vi "FPGAmain_x410_IQ_PID.vi"() -> ()   [LabVIEW 2025]
uses:
  FPGA/DataMode.ctl
  FPGA/Input_5782/5782_Fast_PID_states.ctl
  <vilib>/Platform/TimedLoop/XDataNode/timing_clust.ctl
  <vilib>/Platform/TimedLoop/XDataNode/nitl_modes.ctl
  <vilib>/Platform/TimedLoop/XDataNode/wakeup.ctl
  <vilib>/rvi/Emulation/niFpgaSctlEmulationGetInTimedLoop.vi
  <vilib>/rvi/Emulation/niFpgaEmulationReportErrorSimple.vi
  <vilib>/rvi/Emulation/niFpgaGetClockAttributes.vi
  <vilib>/rvi/Emulation/niFpgaCriticalErrorInLSC.vi
  <vilib>/rvi/Emulation/niFpgaEmulationIsFPGAContextNoSignature.vi
  <vilib>/rvi/DataTransferAndStorage/Container/Common/niFpgaContainerGetUniqueNameForEmu.vi
  <vilib>/rvi/Memory/Memory_Emulation/niFpgaMemoryEmulationCacheClearOnFirstRun.vi
  <vilib>/rvi/Memory/Memory_Emulation/nirvimemoryEmulationManagerCache_MakeExclusive.vi
  <vilib>/rvi/Memory/Memory_Emulation/niFpgaMemoryEmulationValidateCache.vi
  <vilib>/rvi/Memory/Memory_Emulation/nirvimemoryEmulationManagerCache_InsertValue.vi
  <vilib>/Utility/error.llb/Clear Errors.vi
  <vilib>/rvi/Memory/Memory_Emulation/nirvimemoryEmulationManagerCache_ReleaseExclusive.vi
  <vilib>/rvi/Memory/Memory_Emulation/nirvimemoryEmulationManagerCache_GetValue.vi
  <vilib>/rvi/Memory/Memory_Emulation/nirvimemoryEmulationManagerCache_SetValue.vi
  <vilib>/rvi/Emulation/niFpgaProcessEmulError.vi
  <vilib>/rvi/errors/niFpgaSetErrorForExecOnDevCompSimple.vi
  <vilib>/rvi/eio/common/nirviEmuReportErrorAndStop.vi
  <vilib>/rvi/FIFO/Fifo_Resource/nirvififoEmulationSetSize.vi
  <vilib>/rvi/FIFO/Fifo_Resource/nirviFifoEmulationQueueMgr.vi
  <instcachedir>/0/nirviFifoEmulationQueueMgr_E5CAEC123FF24DC58D834DCA3CDAA9B5.lvgen/nirviFifoEmulationQueueMgr_E5CAEC123FF24DC58D834DCA3CDAA9B5_017.vi
  <vilib>/rvi/FIFO/Fifo_Resource/nirvififoEmulationCreateLock.vi
  <vilib>/rvi/FIFO/Fifo_Resource/nirvififoEmulationObtainLock.vi
  <vilib>/rvi/FIFO/Fifo_Resource/nirvififoEmulationReleaseLock.vi
  <vilib>/rvi/occurrence/nirviWaitOnOccurrenceBase.vi
  <vilib>/rvi/errors/nirviReportUnexpectedCaseInternalError.vi
  <vilib>/rvi/errors/nirviReportUnexpectedCaseInternalError (U32).vi
  <instcachedir>/0/nirviFifoEmulationQueueMgr_E5CAEC123FF24DC58D834DCA3CDAA9B5.lvgen/nirviFifoEmulationQueueMgr_E5CAEC123FF24DC58D834DCA3CDAA9B5_004.vi
  <vilib>/rvi/FIFO/Fifo_Resource/nirvififoEmulationDetermineInputValidOut.vi
  <instcachedir>/0/nirviFifoEmulationQueueMgr_E5CAEC123FF24DC58D834DCA3CDAA9B5.lvgen/nirviFifoEmulationQueueMgr_E5CAEC123FF24DC58D834DCA3CDAA9B5_016.vi
  <vilib>/eio/utilities/niEioResolveVilibRelativePath.vi
  <vilib>/rvi/interface/RandomDataEmulation/niFpgaRandomDataHandleErrors.vi
  <instcachedir>/0/nirviFifoEmulationQueueMgr_E5CAEC123FF24DC58D834DCA3CDAA9B5.lvgen/nirviFifoEmulationQueueMgr_E5CAEC123FF24DC58D834DCA3CDAA9B5_006.vi
  <vilib>/rvi/interface/RandomDataEmulation/nirviRandomDataMultiElementFPGAFIFO.vi
  <instcachedir>/0/nirviRandomDataMultiElementFPGAFIFO_BE2FF10D3D6E420AB0291A02835C249E.lvgen/nirviRandomDataMultiElementFPGAFIFO_BE2FF10D3D6E420AB0291A02835C249E_001.vi
  <vilib>/Platform/TimedLoop/XDataNode/XDataNode.xnode
  <vilib>/rvi/DataTransferAndStorage/Container/XNode/niFpgaContainer.xnode
  <vilib>/rvi/DataTransferAndStorage/Register/Emulation/niFpgaRegisterEmulation.vi
  <vilib>/rvi/FIFO/Fifo_Resource/nirvififoEmulationRead.vi
  <vilib>/rvi/FIFO/Fifo_Resource/nirvififoEmulationWrite.vi
  <vilib>/rvi/interface/RandomDataEmulation/nirviRandomDataFpgaReadWriteTemplate.vi
  <vilib>/rvi/interface/RandomDataEmulation/nirviRandomDataFpgaMultiElementTemplate.vi
  <vilib>/eio/EIONode/EIONode.xnode
  <vilib>/rvi/eio/common/nirviEmuTemplateMethod_errors.vi
  <vilib>/Platform/TimedLoop/XDataNode/XDNodeRunTimeDep.lvlib
  <instrlib>/_niInstr/Basic Elements/v1/FPGA/niInstr Basic Elements v1 FPGA.lvlib
panel:
  in  "Output gain":fxp<+/-,16,10>
  out "Amp1":fxp<+,16,14>
  out "TaM":fxp<+/-,32,13>
  out "Quench_Warning":bool
  out "Tau_set":fxp<+/-,32,13>
  in  "Ultra low speed transfer":bool
  out "5782 states":T1
  in  "Full speed transfer":bool
  in  "IO Module\\AO Data Sync":bool=TRUE
  in  "IO Module\\SPI Write Data":u16
  out "IO Module\\SPI Read Data":u8
  in  "IO Module\\SPI Read":bool
  in  "IO Module\\SPI Write":bool
  in  "IO Module\\SPI Address":u16
  in  "IO Module\\SPI Device":u8
  out "IO Module\\SPI Idle":bool
  in  "AM phase":fxp<+,64,64>
  in  "User Command Commit":bool
  in  "User Command":u8
  out "User Command Idle":bool
  out "User Command Status":u8
  in  "User Data 0":u8
  in  "User Data 1":u8
  out "PLL Locked":bool
  out "User Error":bool
  out "Configured?":bool
  in  "Continuous":bool
  in  "Record length":u16=4000 caption="Samples Per Trigger" min=1 step=1
  in  "Trigger Acquisition":bool
  out "IO Module\\Trigger Input":bool
  in  "Acquisition running":bool
  in  "Phase output":fxp<+,64,64>[](array[numeric])=[0.0, 0.0, 0.0, 0.0]
  in  "Simulated phase":fxp<+,64,64>[](array[numeric])=[0.0, 0.0]
  in  "Mode":T2
  in  "Phase input":fxp<+,64,64>[](array[numeric])=[0.0, 0.0, 0.0, 0.0, 0.0, 0.0, 0.0, 0.0, 0.0, 0.0, 0.0, 0.0, 0.0, 0.0, 0.0, 0.0]
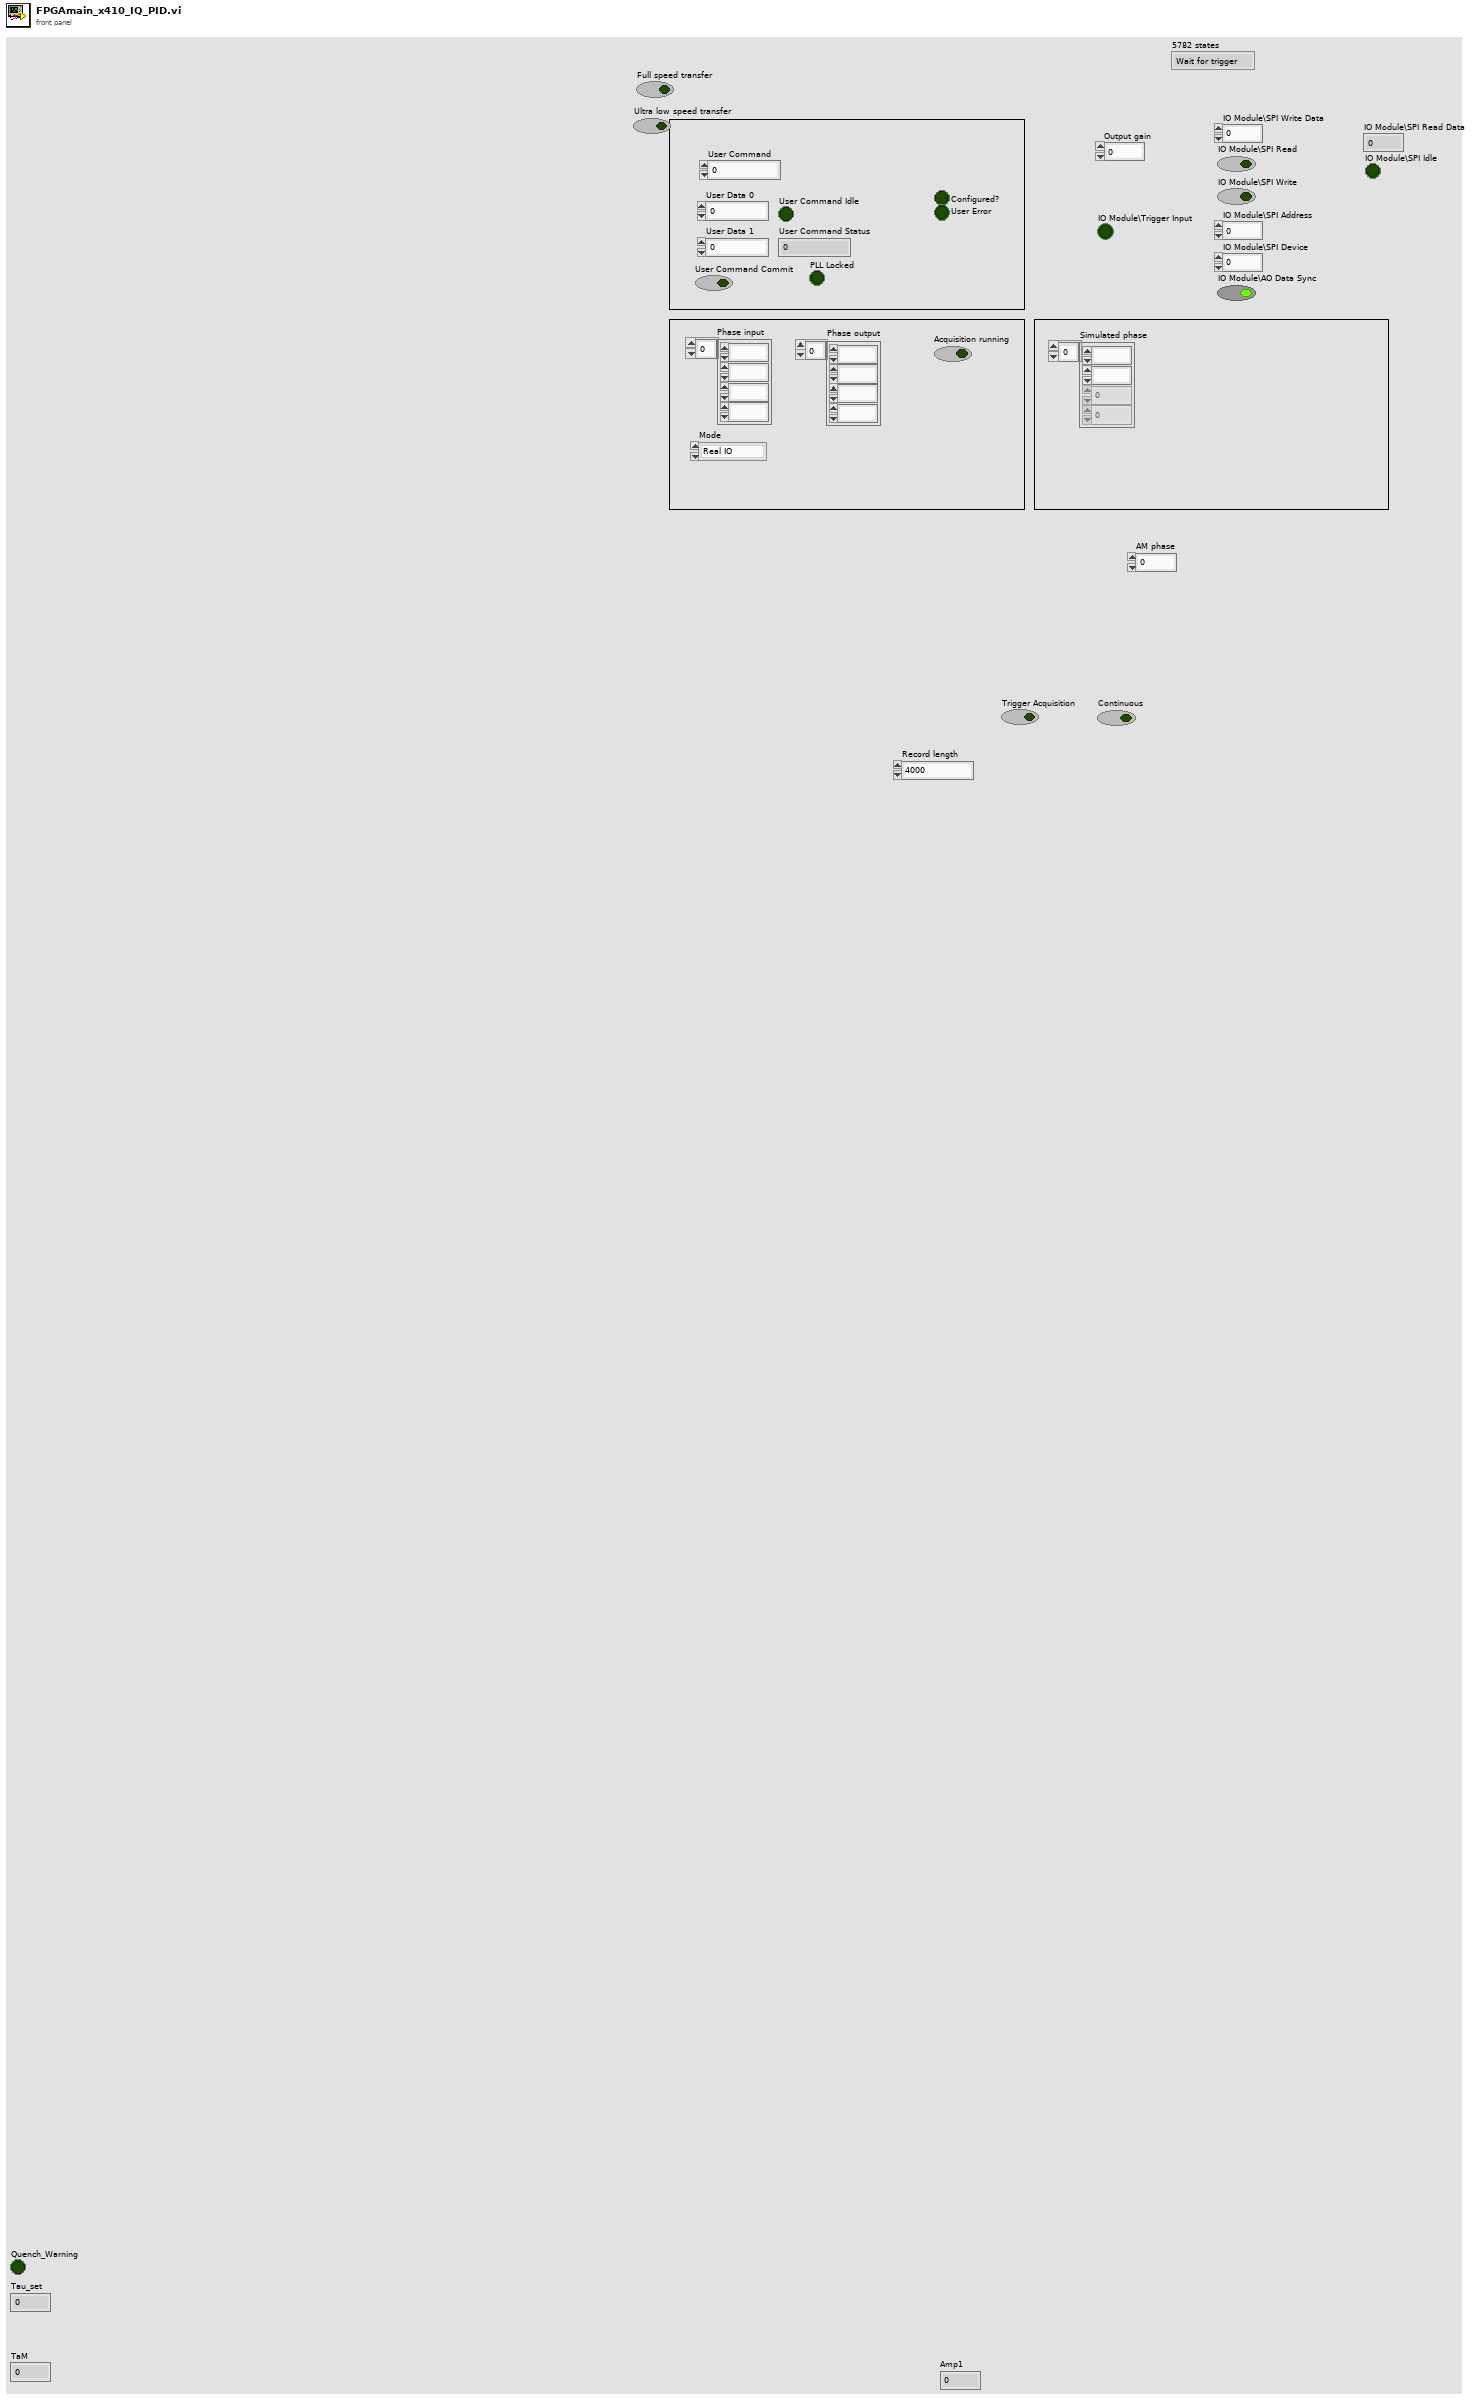
[diagram p1: front panel]
types:
  T1 = typedef "5782_Fast_PID_states.ctl" = enum8{"Wait for trigger", "Acquisition", "Send record length", "Wait for output", "Quiet period"}
  T2 = typedef "DataMode.ctl" = enum16{"Real IO", "Simulated"}
  T3 = typedef "XDNodeRunTimeDep.lvlib/timing_clust.ctl" = cluster{"Expected End [f-1]":u64, "Actual End [f-1]":u64, "Finished Late? [f-1]":bool, "Expected End [i-1]":u64, "Actual End [i-1]":u64, "Finished Late? [i-1]":bool, "Expected Start [i]":u64, "Actual Start [i]":u64, "Expected Start [f]":u64, "Actual Start [f]":u64, "Source Name":string, "Structure Name":string, "Period":i64, "Deadline":i64, "Offset":i64, "Start":i64, "Priority":i32, "Timeout":i32, "Mode":T4, "Wakeup Reason":T5, "Error":errorcluster, "Source Type":string, "Secondary Source Type":string, "Global End Time":u64, "Global Start Time":u64, "Frame Duration":u64, "Iteration Duration":u64, "Assigned CPU":i32, "I/O Scan Engine Mode":u32}
  T4 = typedef "XDNodeRunTimeDep.lvlib/nitl_modes.ctl" = enum32{"No Change", "Process missed periods, maintain original phase", "Discard missed periods, maintain original phase", "Process missed periods, ignore original phase", "Discard missed periods, ignore original phase"}
  T5 = typedef "XDNodeRunTimeDep.lvlib/wakeup.ctl" = enum32{"Normal", "Aborted", "Asynchronous wakeup", "Timing source error", "Timed loop error", "Timeout"}
  T6 = typedef "niInstr DSP v1 Shared.lvlib/IQ Data.ctl" = cluster{"I":fxp<+/-,18,1>, "Q":fxp<+/-,18,1>, "overflow":bool}
  T7 = cluster{"I":fxp<+/-,18,1>, "Q":fxp<+/-,18,1>, "overflow":bool}
  T8 = cluster{"I":fxp<+/-,18,1>, "Q":fxp<+/-,18,1>, "overflow":bool}[]
  T9 = typedef "I32 array size 4.ctl" = fxp<+/-,32,14>[]
  T10 = typedef "IQ-1element.ctl" = T6[]
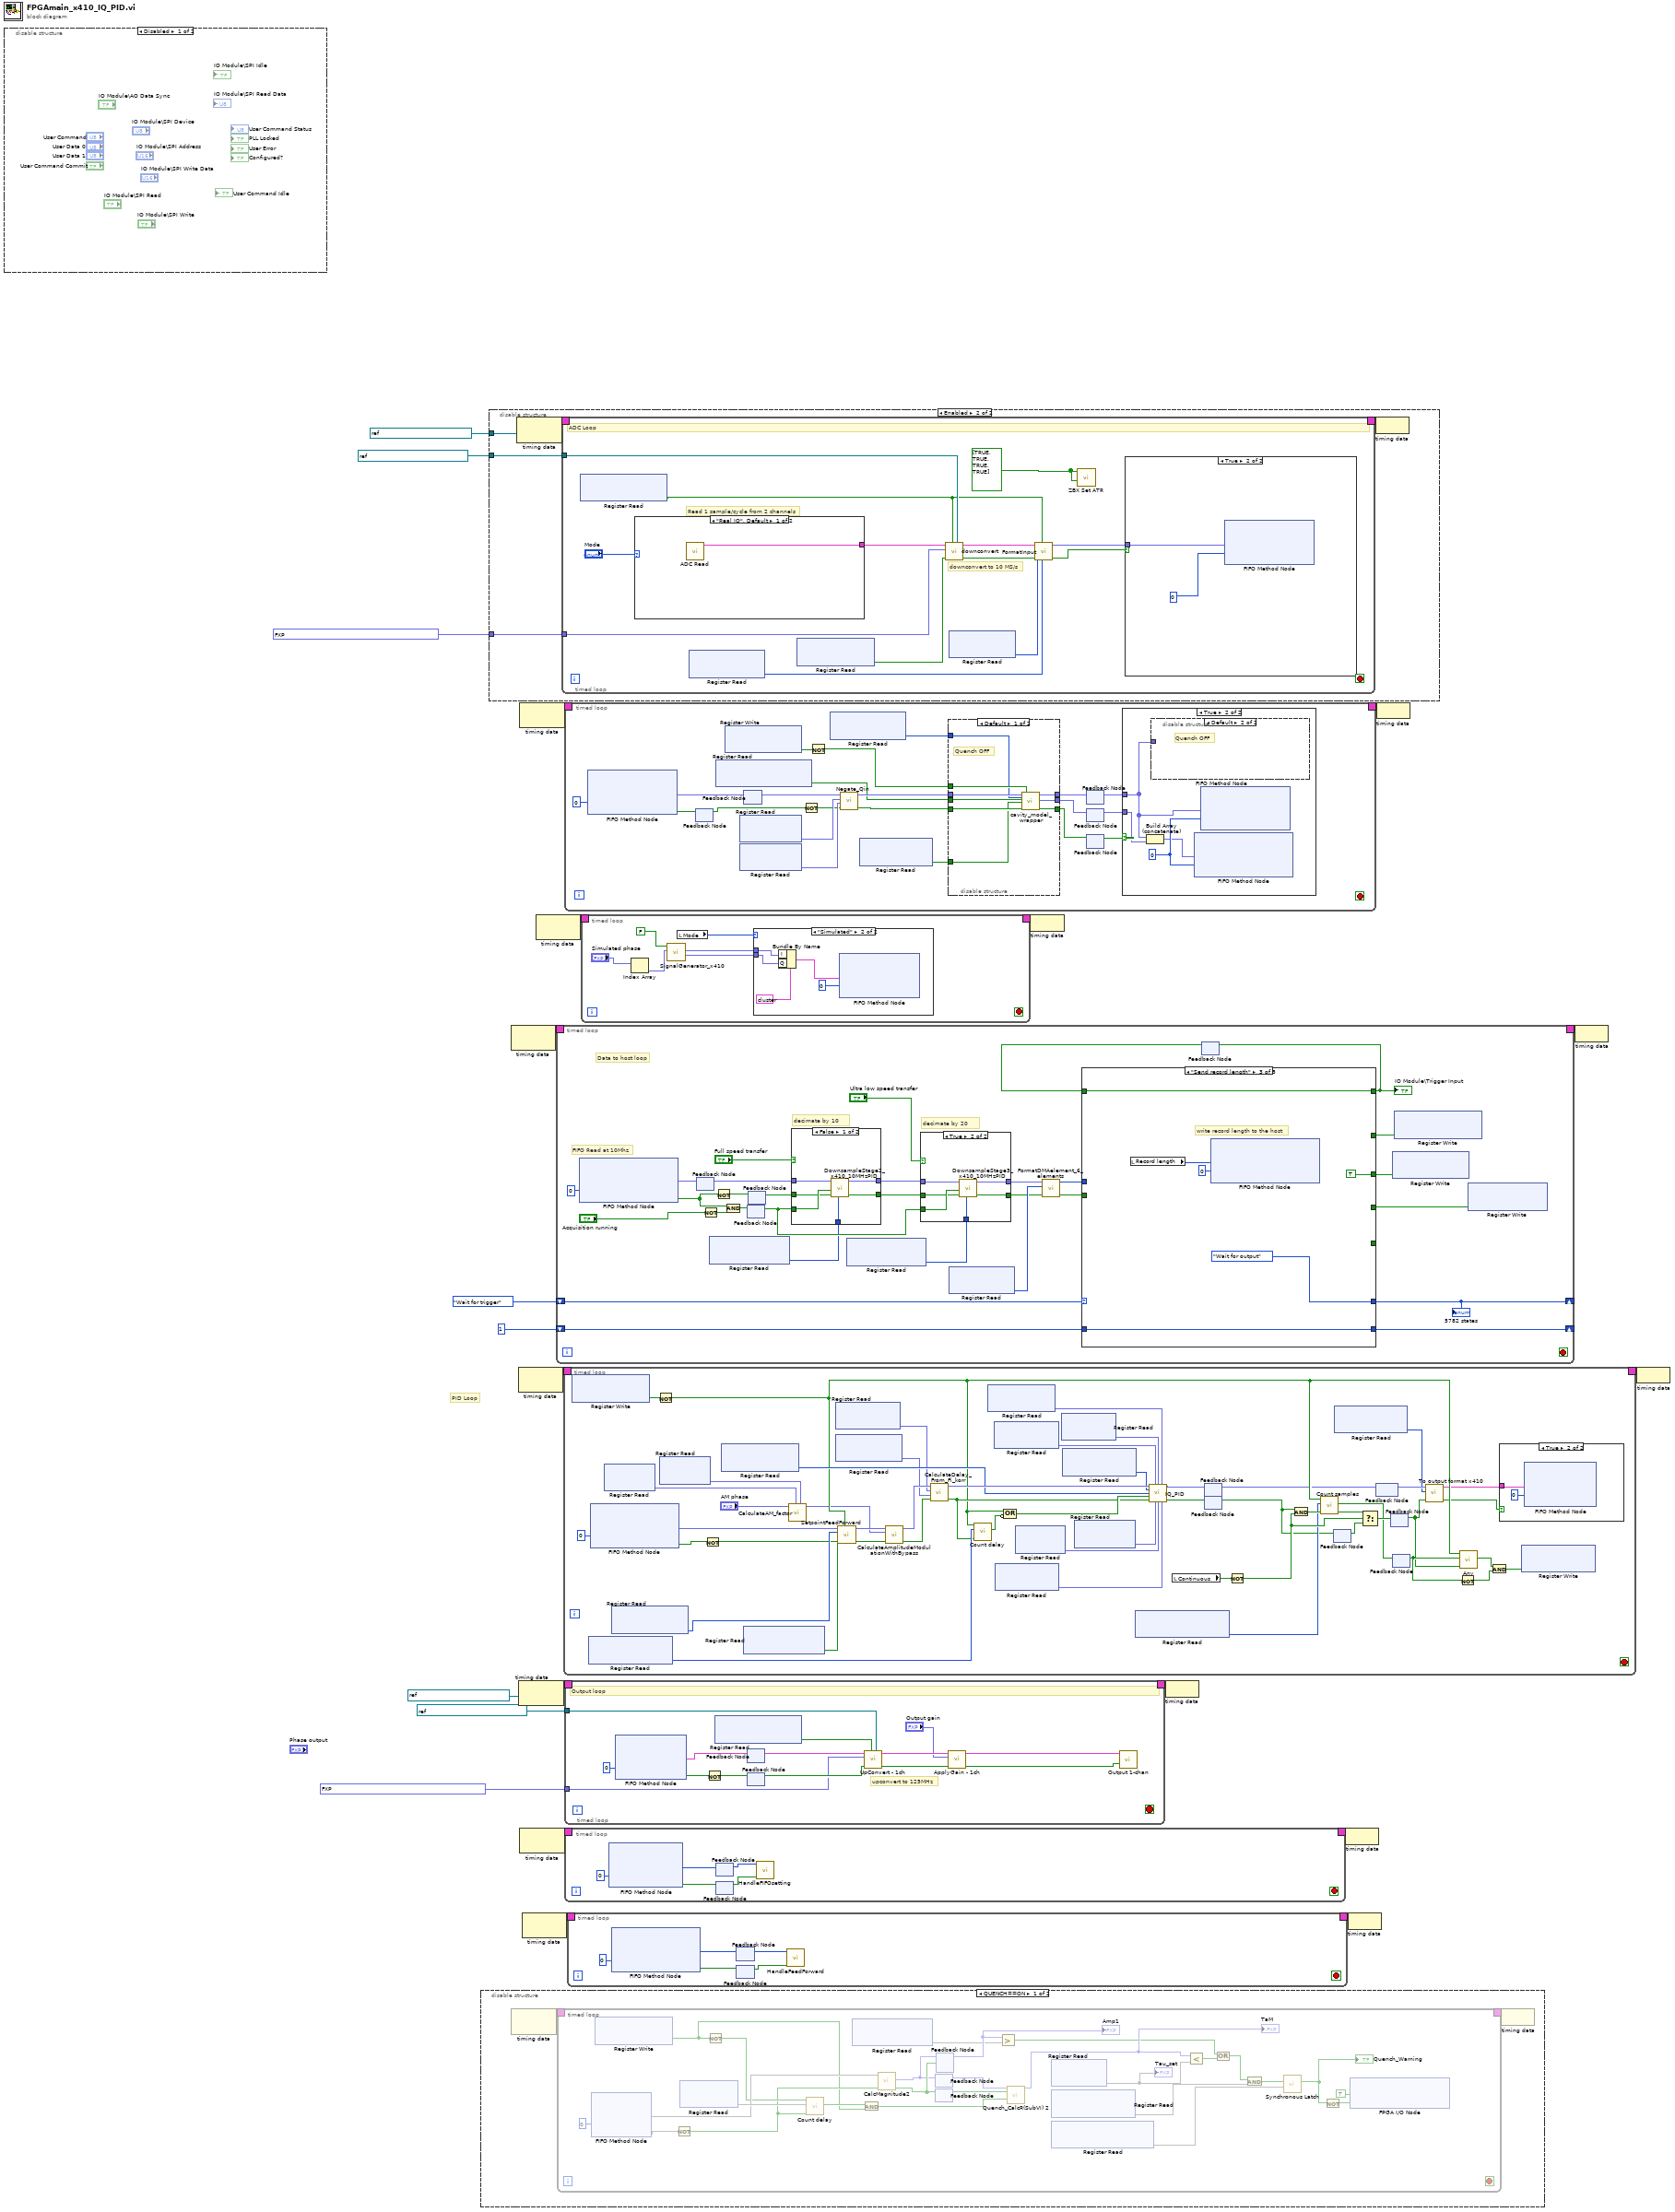
[diagram p0: block diagram]
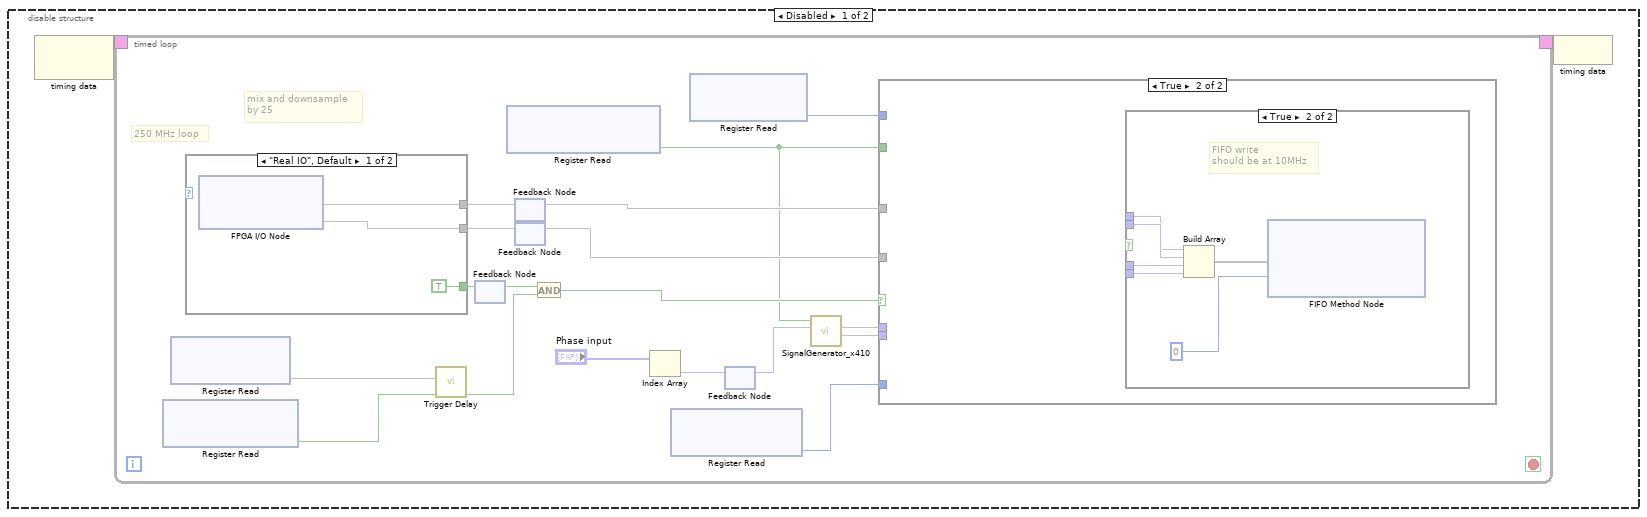
[diagram p2: hidden frame]
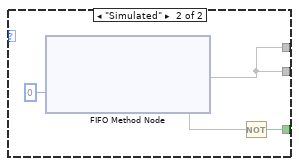
[diagram p5: hidden frame]
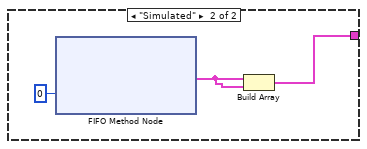
[diagram p6: hidden frame]
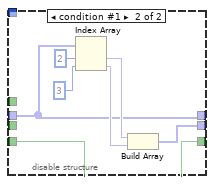
[diagram p11: hidden frame]
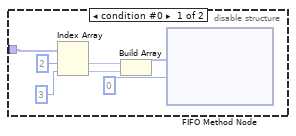
[diagram p13: hidden frame]
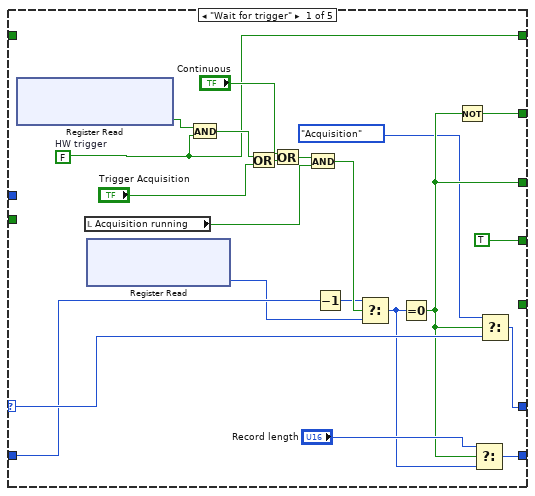
[diagram p16: hidden frame]
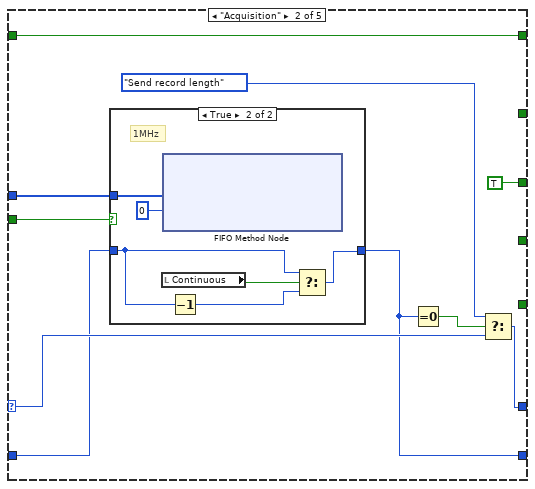
[diagram p17: hidden frame]
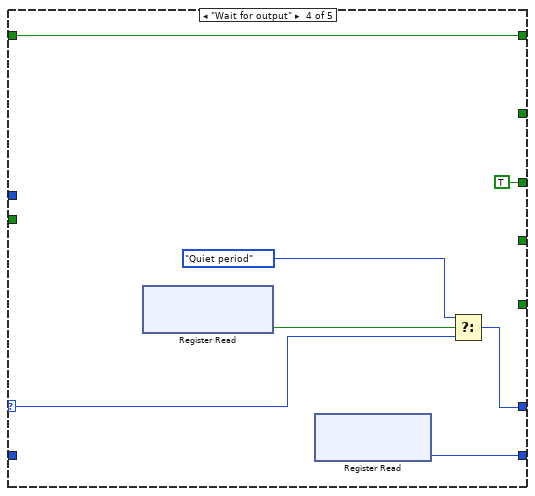
[diagram p19: hidden frame]
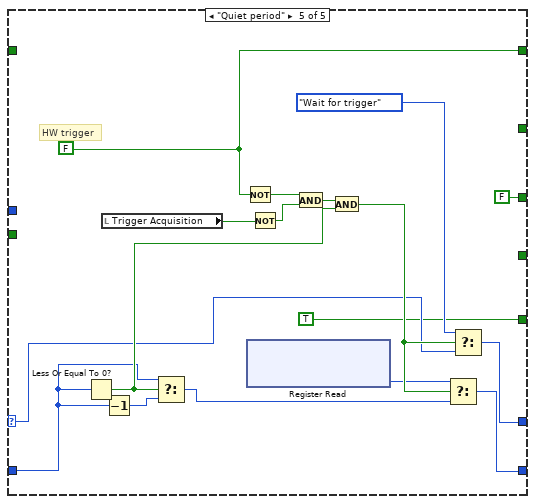
[diagram p20: hidden frame]
diagram:
  # "PID Loop"
  n1 = disable-structure shown="Disabled" {
    frame Disabled {
    }
    frame Enabled {
    }
  }
  n2 = disable-structure shown="QUENCH==ON" {
    frame condition #0 {
      n3 = node-c288() -> (w24:T3)  [unwired: 1 in]
      n4 = timed-loop {
        timing: w24 -> [_]
        timing-out: [_] -> w23
        stop <- _ stop-if-true
        n5 = xnode ("FIFO Method Node")("Timeout"=0) -> ("Element"=w40, "Timed Out?"=w38)  [unwired: 1 in, 1 out]
        n6 = xnode ("Register Write")() -> ("Data"=w34:bool)  [unwired: 1 in, 1 out]
        n7 = Not(x=w38) -> (.not. x?=w37:bool)
        n8 = xnode ("Register Read")() -> ("Data"=w41)  [unwired: 1 in, 1 out]
        n9 = Not(x=w34) -> (.not. x?=w39:bool)
        n10 = call "Count delay.vi"("input valid"=w37, "Count to skip"=w41, "Reset"=w39) -> ("count done?"=w45:bool)  [unwired: 7 in, 1 out]
        n11 = xnode "Register Read"() -> ("Data"=w28)  [unwired: 1 in, 1 out]
        n12 = And(x=w45, y=w34) -> (x .and. y?=w42:bool)
        n13 = call "CalcMagnitude2.vi"("input valid"=w37, "Data in"=w40) -> ("output valid"=w30:bool, "Amp1"=w29:fxp<+,16,14>)  [unwired: 8 in]
        n14 = feedback #1() -> (w44:fxp<+,16,14>)  [unwired: 1 in]
        n15 = feedback-in #1(w29) -> ()
        n16 = feedback #2() -> (w43:bool)  [unwired: 1 in]
        n17 = feedback-in #2(w30) -> ()
        n18 = feedback #3() -> (w31:fxp<+,16,14>)  [unwired: 1 in]
        "Amp1" <- w31
        n19 = feedback-in #3(w29, w30) -> ()
        n20 = Greater?(x=w31, y=w28) -> (0:w25:bool)
        n21 = call "Quench_CalcR(SubVI) 2.vi"("Mag"=w44, "input valid"=w43, "count done?"=w42) -> ("Tau meas"=w35:fxp<+/-,32,13>)  [unwired: 12 in]
        "TaM" <- w35
        n22 = xnode ("Register Read")() -> ("Data"=w49)  [unwired: 1 in, 1 out]
        n23 = xnode ("Register Read")() -> ("Data"=w47)  [unwired: 1 in, 1 out]
        "Tau_set" <- w47
        n24 = xnode ("Register Read")() -> ("Data"=w50)  [unwired: 1 in, 1 out]
        n25 = Less?(x=w35, y=w47) -> (x < y?=w27:bool)
        n26 = Or(x=w25, y=w27) -> (x .or. y?=w26:bool)
        n27 = And(x=w26, y=w50) -> (x .and. y?=w48:bool)
        n28 = call <instrlib>:"Synchronous Latch.vi"("clear"=w49, "set"=w48) -> ("out"=w46:bool)  [unwired: 9 in]
        "Quench_Warning" <- w46
        n29 = Not(x=w46) -> (.not. x?=w33:bool)
        n30 = xnode "FPGA I/O Node"("IO Module\\PFI 2 WE"=TRUE ("IO Module\\PFI 2 WE"), "IO Module\\PFI 2 Wr Data"=w33) -> ()  [unwired: 2 in, 2 out]
      }
      n31 = node-c288(w23) -> ()
    }
    frame condition #1 (active) {
    }
  }
  n32 = disable-structure shown="Enabled" {
    disable-tunnel: fxp<+,48,1> 0.0799999999999983 ("output sample rate") -> [_ w106]
    disable-tunnel: refnum<k21> "Daughterboard 0\\Data Clock x2" ("clock x2") -> [_ w105]
    disable-tunnel: refnum<k21> "Daughterboard 0\\Data Clock" ("Source Name") -> [_ w104]
    frame Disabled {
      n33 = node-c288() -> (w56:T3)  [unwired: 1 in]
      n34 = timed-loop {
        timing: w56 -> [_]
        timing-out: [_] -> w55
        stop <- _ stop-if-true
        # "mix and downsample\nby 25"
        # "250 MHz loop"
        n35 = xnode ("Register Read")() -> ("Data"=w62:bool)  [unwired: 1 in, 1 out]
        n36 = xnode ("Register Read")() -> ("Data"=w60)  [unwired: 1 in, 1 out]
        n37 = case shown="\"Real IO\", Default" {
          selector: _ -> [_ _]
          tunnel: [w95 w96] -> w74
          tunnel: [w94 w96] -> w72
          tunnel: [TRUE w97] -> w70
          frame "Real IO", Default {
            n38 = xnode "FPGA I/O Node"() -> ("IO Module\\AI 0"=w95, "IO Module\\AI 1"=w94)  [unwired: 2 in, 2 out]
          }
          frame "Simulated" {
            n39 = xnode ("FIFO Method Node")("Timeout"=0) -> ("Element"=w96, "Timed Out?"=w98)  [unwired: 1 in, 1 out]
            n40 = Not(x=w98) -> (.not. x?=w97:bool)
          }
        }
        n41 = call "Trigger Delay.vi"("input valid"=w62, "Count to skip"=w60) -> ("output valid"=w61:bool)  [unwired: 9 in]
        n42 = feedback #4() -> (w69:bool)  [unwired: 1 in]
        n43 = feedback-in #4(w70) -> ()
        n44 = xnode ("Register Read")() -> ("Data"=w58:bool)  [unwired: 1 in, 1 out]
        n45 = feedback #5() -> (w73)  [unwired: 1 in]
        n46 = feedback-in #5(w74) -> ()
        n47 = feedback #6() -> (w71)  [unwired: 1 in]
        n48 = feedback-in #6(w72) -> ()
        n49 = And(x=w69, y=w61) -> (x .and. y?=w66:bool)
        n50 = Index Array(array="Phase input") -> (element=w64:fxp<+,64,64>)  [unwired: 1 in]
        n51 = xnode ("Register Read")() -> ("Data"=w57:u32)  [unwired: 1 in, 1 out]
        n52 = xnode ("Register Read")() -> ("Data"=w59:u16)  [unwired: 1 in, 1 out]
        n53 = feedback #7() -> (w63:fxp<+,64,64>)  [unwired: 1 in]
        n54 = feedback-in #7(w64) -> ()
        n55 = call "SignalGenerator_x410.vi"("phase"=w63, "Reset"=w58) -> ("Cos"=w68:fxp<+/-,18,1>, "Sin"=w67:fxp<+/-,18,1>)  [unwired: 7 in, 1 out]
        n56 = case shown="True" w66 {
          tunnel: w73 -> [_ w86]
          tunnel: w71 -> [_ w85]
          tunnel: w68 -> [_ w79]
          tunnel: w67 -> [_ w78]
          tunnel: w59 -> [_ w77]
          tunnel: w58 -> [_ w76]
          tunnel: w57 -> [_ w75]
          frame False {
          }
          frame True {
            n57 = case shown="True" w82 {
              tunnel: [_ w92] -> w83
              tunnel: [_ w91] -> w84
              tunnel: [_ w90] -> w81
              tunnel: [_ w89] -> w80
              frame False {
              }
              frame True {
                # "FIFO write\nshould be at 10MHz"
                n58 = Build Array(w91, w92, w90, w89) -> (w88:void[])
                n59 = xnode ("FIFO Method Node")("Element"=w88, "Timeout"=0) -> ()  [unwired: 1 in, 2 out]
              }
            }
          }
        }
      }
      n60 = node-c288(w55) -> ()
    }
    frame Enabled {
      n61 = node-c288(w104) -> (w108:T3)
      n62 = timed-loop "Acquisition Loop" {
        timing: w108 -> [_]
        timing-out: [_] -> w107
        tunnel: w106 -> [w121]
        tunnel: w105 -> [w118]
        stop <- _ stop-if-true
        w119 = bool[] [TRUE, TRUE, TRUE, TRUE] ("DB 0")
        # "Read 1 sample/cycle from 2 channels"
        # "downconvert to 10 MS/s"
        # "ADC Loop"
        n63 = xnode ("Register Read")() -> ("Data"=w113:bool)  [unwired: 1 in, 1 out]
        n64 = case shown="\"Real IO\", Default" "Mode" {
          tunnel: [w122 w124] -> w120
          frame "Real IO", Default {
            n65 = call "ADC Read.vi"() -> ("Data out"=w122:T6[])  [unwired: 11 in]
          }
          frame "Simulated" {
            n66 = xnode ("FIFO Method Node")("Timeout"=0) -> ("Element"=w125:T7)  [unwired: 1 in, 2 out]
            n67 = Build Array(w125, w125) -> (w124:T8)
          }
        }
        n68 = xnode ("Register Read")() -> ("Data"=w114:u32)  [unwired: 1 in, 1 out]
        n69 = xnode ("Register Read")() -> ("Data"=w112:bool)  [unwired: 1 in, 1 out]
        n70 = call "downconvert.vi"("clock x2"=w118, "reset"=w113, "input valid"=w112, "output sample rate"=w121, "data in"=w120) -> ("output valid"=w111:bool, "data out"=w116:T6[])  [unwired: 5 in]
        n71 = xnode ("Register Read")() -> ("Data"=w109:u16)  [unwired: 1 in, 1 out]
        n72 = call "FormatInput.vi"("Count to skip"=w114, "reset"=w113, "valid in"=w111, "factor"=w109, "data in"=w116) -> ("valid out"=w110:bool, "Array out"=w115:T9)  [unwired: 5 in]
        n73 = call <instrlib>:"ZBX Set ATR.vi"("DB 1"=w119, "DB 0"=w119) -> ()  [unwired: 10 in]
        n74 = case shown="True" w110 {
          tunnel: w115 -> [_ w126]
          frame False {
          }
          frame True {
            n75 = xnode ("FIFO Method Node")("Element"=w126, "Timeout"=0) -> ()  [unwired: 1 in, 2 out]
          }
        }
      }
      n76 = node-c288(w107) -> ()
    }
  }
  n77 = node-c288() -> (w17:T3)  [unwired: 1 in]
  n78 = node-c288() -> (w19:T3)  [unwired: 1 in]
  n79 = node-c288(refnum<k21> "Daughterboard 0\\Data Clock" ("Source Name")) -> (w5:T3)
  n80 = node-c288() -> (w12:T3)  [unwired: 1 in]
  n81 = node-c288() -> (w21:T3)  [unwired: 1 in]
  n82 = node-c288() -> (w14:T3)  [unwired: 1 in]
  n83 = node-c288() -> (w10:T3)  [unwired: 1 in]
  n84 = timed-loop {
    timing: w17 -> [_]
    timing-out: [_] -> w16
    shift-right: [w161] -> _
    shift-left: 5782_Fast_PID_states."Wait for trigger" ("5782 states") -> [w163]
    shift-right: [w160] -> _
    shift-left: u16 1 ("trigger samples") -> [w162]
    stop <- _ stop-if-true
    # "decimate by 20"
    # "Data to host loop"
    # "FIFO Read at 10Mhz"
    # "decimate by 10"
    n85 = xnode ("FIFO Method Node")("Timeout"=0) -> ("Element"=w144:fxp<+/-,32,14>[], "Timed Out?"=w143:bool)  [unwired: 1 in, 1 out]
    n86 = feedback #8() -> (w145:fxp<+/-,32,14>[])  [unwired: 1 in]
    n87 = feedback-in #8(w144) -> ()
    n88 = Not(x="Acquisition running") -> (.not. x?=w150:bool)
    n89 = xnode ("Register Read")() -> ("Data"=w135:u32)  [unwired: 1 in, 1 out]
    n90 = Not(x=w143) -> (.not. x?=w148:bool)
    n91 = And(x=w143, y=w150) -> (x .and. y?=w147:bool)
    n92 = feedback #9() -> (w140:bool)  [unwired: 1 in]
    n93 = feedback-in #9(w147) -> ()
    n94 = feedback #10() -> (w149:bool)  [unwired: 1 in]
    n95 = feedback-in #10(w148) -> ()
    n96 = case shown="False" "Full speed transfer" {
      tunnel: [w177 w179] -> w138
      tunnel: [w176 w178] -> w139
      tunnel: w145 -> [w175 w179]
      tunnel: w140 -> [w174 _]
      tunnel: w149 -> [w173 w178]
      tunnel: w135 -> [w172 _]
      frame False {
        n97 = call "DownsampleStage2_x410_10MHzPID.vi"("Count to skip"=w172, "valid in"=w173, "reset"=w174, "Data in"=w175) -> ("valid out"=w176:bool, "data out"=w177:fxp<+/-,32,14>[])  [unwired: 6 in]
      }
      frame True {
      }
    }
    n98 = xnode ("Register Read")() -> ("Data"=w134:u32)  [unwired: 1 in, 1 out]
    n99 = case shown="True" "Ultra low speed transfer" {
      tunnel: [w165 w170] -> w136
      tunnel: [w164 w169] -> w137
      tunnel: w138 -> [w165 w171]
      tunnel: w140 -> [_ w168]
      tunnel: w139 -> [w164 w167]
      tunnel: w134 -> [_ w166]
      frame False {
      }
      frame True {
        n100 = call "DownsampleStage3_x410_10MHzPID.vi"("Count to skip"=w166, "valid in"=w167, "reset"=w168, "Data in"=w171) -> ("valid out"=w169:bool, "data out"=w170:fxp<+/-,32,14>[])  [unwired: 6 in]
      }
    }
    n101 = xnode ("Register Read")() -> ("Data"=w153:u16)  [unwired: 1 in, 1 out]
    n102 = call "FormatDMAelement_6_elements.vi"("valid in"=w137, "factor"=w153, "Data in"=w136) -> ("valid out"=w156:bool, "Values"=w155:u64[])  [unwired: 7 in]
    n103 = feedback #11() -> (w158:bool)  [unwired: 1 in]
    n104 = case shown="\"Send record length\"" w163 {
      selector: w163 -> [w200 w210 _ w228 w235]
      tunnel: w162 -> [w191 w207 w220 _ w236]
      tunnel: [w199 w209 5782_Fast_PID_states."Wait for output" ("5782 states") w230 w246] -> w161
      tunnel: [w198 w204 w220 w226 w247] -> w160
      tunnel: w155 -> [_ w205 _ _ _]
      tunnel: w156 -> [_ w206 _ _ _]
      tunnel: [w186 TRUE TRUE ("5782 triggered") TRUE ("5782 triggered") FALSE ("5782 triggered")] -> w159
      tunnel: [w180 w203 w222 w225 w231] -> w157
      tunnel: w158 -> [_ w203 w222 w225 _]
      tunnel: [w185 _ _ _ _] -> w154
      tunnel: [TRUE _ _ _ _] -> w152
      tunnel: [_ _ _ _ TRUE ("5782 triggered")] -> _
      frame "Wait for trigger" {
        w180 = FALSE  # HW trigger
        n105 = xnode ("Register Read")() -> ("Data"=w182:bool)  [unwired: 1 in, 1 out]
        n106 = local read "Acquisition running"() -> (w194:bool)
        n107 = xnode ("Register Read")() -> ("Data"=w187:u16)  [unwired: 1 in, 1 out]
        n108 = And(x=w182, y=w180) -> (x .and. y?=w181:bool)
        n109 = Or(x=w181, y="Trigger Acquisition") -> (x .or. y?=w190:bool)
        n110 = Or(x="Continuous", y=w190) -> (x .or. y?=w188:bool)
        n111 = And(x=w188, y=w194) -> (x .and. y?=w195:bool)
        n112 = Decrement(x=w191) -> (x-1=w192:u16)
        n113 = Select(t=w192, s=w195, f=w187) -> (s? t:f=w193:u16)
        n114 = Equal To 0?(x=w193) -> (x = 0?=w186:bool)
        n115 = Not(x=w186) -> (.not. x?=w185:bool)
        n116 = Select(t="Record length", s=w186, f=w193) -> (s? t:f=w198:u16)
        n117 = Select(t=5782_Fast_PID_states."Acquisition" ("5782 states"), s=w186, f=w200) -> (s? t:f=w199:T1)
      }
      frame "Acquisition" {
        n118 = case shown="True" w206 {
          tunnel: w205 -> [_ w217]
          tunnel: [w211 w214] -> w204
          tunnel: w207 -> [w211 w212]
          frame False {
          }
          frame True {
            # "1MHz"
            n119 = local read "Continuous"() -> (w215:bool)
            n120 = xnode ("FIFO Method Node")("Element"=w217, "Timeout"=0) -> ()  [unwired: 1 in, 2 out]
            n121 = Decrement(x=w212) -> (x-1=w213:u16)
            n122 = Select(t=w212, s=w215, f=w213) -> (s? t:f=w214:u16)
          }
        }
        n123 = Equal To 0?(x=w204) -> (x = 0?=w208:bool)
        n124 = Select(t=5782_Fast_PID_states."Send record length" ("5782 states"), s=w208, f=w210) -> (s? t:f=w209:T1)
      }
      frame "Send record length" {
        # "write record length to the host"
        n125 = local read "Record length"() -> (w219:u16)
        n126 = xnode ("FIFO Method Node")("Element"=w219, "Timeout"=0) -> ()  [unwired: 1 in, 2 out]
      }
      frame "Wait for output" {
        n127 = xnode ("Register Read")() -> ("Data"=w224:bool)  [unwired: 1 in, 1 out]
        n128 = xnode ("Register Read")() -> ("Data"=w226:u16)  [unwired: 1 in, 1 out]
        n129 = Select(t=5782_Fast_PID_states."Quiet period" ("5782 states"), s=w224, f=w228) -> (s? t:f=w230:T1)
      }
      frame "Quiet period" {
        w231 = FALSE ("5782 triggered")
        # "HW trigger"
        n130 = Less Or Equal To 0?(x=w236) -> (x <= 0?=w239:bool)
        n131 = local read "Trigger Acquisition"() -> (w244:bool)
        n132 = Decrement(x=w236) -> (x-1=w240:u16)
        n133 = Select(t=w236, s=w239, f=w240) -> (s? t:f=w238:u16)
        n134 = Not(x=w231) -> (.not. x?=w233:bool)
        n135 = xnode ("Register Read")() -> ("Data"=w237:u16)  [unwired: 1 in, 1 out]
        n136 = Not(x=w244) -> (.not. x?=w243:bool)
        n137 = And(x=w233, y=w243) -> (x .and. y?=w242:bool)
        n138 = And(x=w242, y=w239) -> (x .and. y?=w245:bool)
        n139 = Select(t=w237, s=w245, f=w238) -> (s? t:f=w247:u16)
        n140 = Select(t=5782_Fast_PID_states."Wait for trigger" ("5782 states"), s=w245, f=w235) -> (s? t:f=w246:T1)
      }
    }
    "IO Module\\Trigger Input" <- w157
    "5782 states" <- w161
    n141 = feedback-in #11(w157) -> ()
    n142 = xnode ("Register Write")("Data"=w159) -> ()  [unwired: 1 in, 1 out]
    n143 = xnode ("Register Write")("Data"=w154) -> ()  [unwired: 1 in, 1 out]
    n144 = xnode ("Register Write")("Data"=w152) -> ()  [unwired: 1 in, 1 out]
  }
  n145 = timed-loop {
    timing: w19 -> [_]
    timing-out: [_] -> w18
    stop <- _ stop-if-true
    n146 = xnode ("Register Write")() -> ("Data"=w299:bool)  [unwired: 1 in, 1 out]
    n147 = xnode ("Register Read")() -> ("Data"=w295:u32)  [unwired: 1 in, 1 out]
    n148 = xnode ("FIFO Method Node")("Timeout"=0) -> ("Element"=w293:fxp<+/-,32,14>[], "Timed Out?"=w300:bool)  [unwired: 1 in, 1 out]
    n149 = xnode ("Register Read")() -> ("Data"=w259:fxp<+/-,16,2>)  [unwired: 1 in, 1 out]
    n150 = xnode ("Register Read")() -> ("Data"=w294:u32)  [unwired: 1 in, 1 out]
    n151 = Not(x=w299) -> (.not. x?=w266:bool)
    n152 = xnode ("Register Read")() -> ("Data"=w258:fxp<+/-,16,2>)  [unwired: 1 in, 1 out]
    n153 = Not(x=w300) -> (.not. x?=w292:bool)
    n154 = xnode ("Register Read")() -> ("Data"=w283:enum16{"PID on", "Ref", "Zero"})  [unwired: 1 in, 1 out]
    n155 = xnode ("Register Read")() -> ("Data"=w298:bool)  [unwired: 1 in, 1 out]
    n156 = call "CalculateAM_factor.vi"("b_am"=w258, "a_am"=w259, "AM phase"="AM phase") -> ("AM_factor"=w261:fxp<+/-,16,2>)  [unwired: 7 in, 1 out]
    n157 = xnode ("Register Read")() -> ("Data"=w252:fxp<+/-,16,2>)  [unwired: 1 in, 1 out]
    n158 = xnode ("Register Read")() -> ("Data"=w253:fxp<+/-,16,2>)  [unwired: 1 in, 1 out]
    n159 = call "SetpointFeedForward.vi"("Reset"=w266, "input valid"=w292, "setpoint enabled"=w298, "Samples to skip"=w294, "Data in"=w293) -> ("output valid"=w255:bool, "Data out"=w263:fxp<+/-,32,14>[])  [unwired: 5 in]
    n160 = call "CalculateAmplitudeModulationWithBypass.vi"("input valid"=w255, "AM_factor"=w261, "Data in"=w263) -> ("output valid"=w254:bool, "Data out"=w262:fxp<+/-,32,14>[])  [unwired: 7 in]
    n161 = call "CalculateDelay_From_Fi_korr.vi"("input valid"=w254, "cos(x)"=w253, "sin(x)"=w252, "Data in"=w262) -> ("output valid"=w284:bool, "Data out"=w291:fxp<+/-,32,14>[])  [unwired: 6 in]
    n162 = call "Count delay.vi"("input valid"=w284, "Count to skip"=w295, "Reset"=w266) -> ("count done?"=w296:bool)  [unwired: 7 in, 1 out]
    n163 = xnode ("Register Read")() -> ("Data"=w286:fxp<+/-,32,11>)  [unwired: 1 in, 1 out]
    n164 = xnode ("Register Read")() -> ("Data"=w289:fxp<+/-,32,6>)  [unwired: 1 in, 1 out]
    n165 = xnode ("Register Read")() -> ("Data"=w280:fxp<+/-,32,11>)  [unwired: 1 in, 1 out]
    n166 = Compound Arithmetic op=OR(w266, invert w296) -> (w285:bool)
    n167 = xnode ("Register Read")() -> ("Data"=w281:fxp<+/-,32,6>)  [unwired: 1 in, 1 out]
    n168 = xnode ("Register Read")() -> ("Data"=w288:fxp<+/-,32,6>)  [unwired: 1 in, 1 out]
    n169 = xnode ("Register Read")() -> ("Data"=w290:enum16{"PID on", "Ref", "Zero"})  [unwired: 1 in, 1 out]
    n170 = xnode ("Register Read")() -> ("Data"=w282:fxp<+/-,32,6>)  [unwired: 1 in, 1 out]
    n171 = xnode ("Register Read")() -> ("Data"=w270:u32)  [unwired: 1 in, 1 out]
    n172 = call "IQ_PID.vi"("Data in"=w291, "Ki*Tau I"=w289, "Kp I"=w288, "Kd/Tau I"=w286, "Enable I"=w290, "Enable Q"=w283, "Reset"=w285, "input valid"=w284, "Ki*Tau Q"=w282, "Kp Q"=w281, "Kd/Tau Q"=w280) -> ("data out"=w287:fxp<+/-,32,14>[], "output valid"=w264:bool)  [unwired: 1 in, 2 out]
    n173 = local read "Continuous"() -> (w279:bool)
    n174 = feedback #12() -> (w257:fxp<+/-,32,14>[])  [unwired: 1 in]
    n175 = feedback-in #12(w287) -> ()
    n176 = feedback #13() -> (w256:bool)  [unwired: 1 in]
    n177 = feedback-in #13(w264) -> ()
    n178 = Not(x=w279) -> (.not. x?=w272:bool)
    n179 = And(x=w256, y=w272) -> (x .and. y?=w274:bool)
    n180 = call "Count samples.vi"("input valid"=w274, "number to count"=w270, "Reset"=w266) -> ("output valid"=w275:bool, "counting"=w271:bool)  [unwired: 7 in]
    n181 = feedback #14() -> (w273:bool)  [unwired: 1 in]
    n182 = feedback-in #14(w256) -> ()
    n183 = xnode ("Register Read")() -> ("Data"=w267:u16)  [unwired: 1 in, 1 out]
    n184 = Select(t=w275, s=w272, f=w273) -> (s? t:f=w276:bool)
    n185 = feedback #15() -> (w269:fxp<+/-,32,14>[])  [unwired: 1 in]
    n186 = feedback-in #15(w257) -> ()
    n187 = feedback-in #16(w276) -> ()
    n188 = feedback #16() -> (w268:bool)  [unwired: 1 in]
    n189 = feedback #17() -> (w278:bool)  [unwired: 1 in]
    n190 = feedback-in #17(w271) -> ()
    n191 = call "To output format x410.vi"("input valid"=w268, "factor"=w267, "Data in"=w269) -> ("output valid"=w251:bool, "Data out"=w250:T10)  [unwired: 7 in]
    n192 = Not(x=w278) -> (.not. x?=w277:bool)
    n193 = call "Any.vi"("input valid"=w268, "Value"=w278, "Reset"=w266) -> ("Any?"=w265:bool)  [unwired: 7 in, 1 out]
    n194 = And(x=w265, y=w277) -> (x .and. y?=w297:bool)
    n195 = case shown="True" w251 {
      tunnel: w250 -> [_ w303]
      frame False {
      }
      frame True {
        n196 = xnode ("FIFO Method Node")("Element"=w303, "Timeout"=0) -> ()  [unwired: 1 in, 2 out]
      }
    }
    n197 = xnode ("Register Write")("Data"=w297) -> ()  [unwired: 1 in, 1 out]
  }
  n198 = timed-loop "Acquisition Loop" {
    timing: w5 -> [_]
    timing-out: [_] -> w4
    tunnel: refnum<k21> "Daughterboard 0\\Data Clock x2" ("clock x2") -> [w313]
    tunnel: fxp<+,48,1> 0.0799999999999983 ("output sample rate") -> [w312]
    stop <- _ stop-if-true
    # "upconvert to 125MHz"
    # "Output loop"
    n199 = xnode ("FIFO Method Node")("Timeout"=0) -> ("Element"=w318:T8, "Timed Out?"=w319:bool)  [unwired: 1 in, 1 out]
    n200 = Not(x=w319) -> (.not. x?=w317:bool)
    n201 = xnode ("Register Read")() -> ("Data"=w311:bool)  [unwired: 1 in, 1 out]
    n202 = feedback #18() -> (w315:bool)  [unwired: 1 in]
    n203 = feedback-in #18(w317) -> ()
    n204 = feedback #19() -> (w314:T8)  [unwired: 1 in]
    n205 = feedback-in #19(w318) -> ()
    n206 = call "UpConvert - 1ch.vi"("clock x2"=w313, "reset"=w311, "input valid"=w315, "output sample rate"=w312, "data in"=w314) -> ("output valid"=w308:bool, "data out"=w310:T10)  [unwired: 5 in]
    n207 = call "ApplyGain - 1ch.vi"("input valid"=w308, "gain"="Output gain", "data in"=w310) -> ("output valid"=w307:bool, "data out"=w309:T6[])  [unwired: 7 in]
    n208 = call "Output 1-chan.vi"("data"=w309, "input valid"=w307) -> ()  [unwired: 14 in]
  }
  n209 = timed-loop {
    timing: w12 -> [_]
    timing-out: [_] -> w11
    stop <- _ stop-if-true
    n210 = xnode ("FIFO Method Node")("Timeout"=0) -> ("Element"=w328:fxp<+/-,32,14>[], "Timed Out?"=w327:bool)  [unwired: 1 in, 1 out]
    n211 = feedback #20() -> (w325:bool)  [unwired: 1 in]
    n212 = feedback-in #20(w327) -> ()
    n213 = xnode ("Register Read")() -> ("Data"=w336:bool)  [unwired: 1 in, 1 out]
    n214 = xnode ("Register Write")() -> ("Data"=w335:bool)  [unwired: 1 in, 1 out]
    n215 = xnode ("Register Read")() -> ("Data"=w341:fxp<+/-,32,14>)  [unwired: 1 in, 1 out]
    n216 = xnode ("Register Read")() -> ("Data"=w342:fxp<+/-,32,14>)  [unwired: 1 in, 1 out]
    n217 = feedback #21() -> (w326:fxp<+/-,32,14>[])  [unwired: 1 in]
    n218 = feedback-in #21(w328) -> ()
    n219 = Not(x=w325) -> (.not. x?=w340:bool)
    n220 = Not(x=w335) -> (.not. x?=w337:bool)
    n221 = xnode ("Register Read")() -> ("Data"=w322:enum16{"Off", "On - Ch 0", "On - Ch 1"})  [unwired: 1 in, 1 out]
    n222 = call "Negate_Qin.vi"("valid in"=w340, "DC offset chan 1"=w341, "DC offset chan 0"=w342, "Data in"=w326) -> ("valid out"=w338:bool, "Data out"=w339:fxp<+/-,32,14>[])  [unwired: 6 in]
    n223 = xnode ("Register Read")() -> ("Data"=w323:bool)  [unwired: 1 in, 1 out]
    n224 = disable-structure shown="Default" {
      disable-tunnel: w339 -> [w351 w353]
      disable-tunnel: w338 -> [w350 w358]
      disable-tunnel: w337 -> [w349 _]
      disable-tunnel: w336 -> [w348 _]
      disable-tunnel: [w347 w353] -> w334
      disable-tunnel: [w346 w358] -> w332
      disable-tunnel: [w345 w352] -> w330
      disable-tunnel: w323 -> [w344 _]
      disable-tunnel: w322 -> [w343 _]
      frame condition #0 (active) {
        # "Quench OFF"
        n225 = call "cavity_model_wrapper.vi"("Data in"=w351, "Piezo setting"=w343, "enabled"=w348, "virtual cavity"=w344, "input valid"=w350, "reset"=w349) -> ("Data out"=w347:fxp<+/-,32,14>[], "Ai1 out"=w345:fxp<+/-,32,14>[], "output valid"=w346:bool)  [unwired: 11 in]
      }
      frame condition #1 {
        n226 = Index Array(array=w353, index #1=2 ("index"), index #2=3 ("index")) -> (element #1=w357:fxp<+/-,32,14>, element #2=w356:fxp<+/-,32,14>)
        n227 = Build Array(w357, w356) -> (w352:fxp<+/-,32,14>[])
      }
    }
    n228 = feedback #22() -> (w333:fxp<+/-,32,14>[])  [unwired: 1 in]
    n229 = feedback-in #22(w334) -> ()
    n230 = feedback #23() -> (w329:fxp<+/-,32,14>[])  [unwired: 1 in]
    n231 = feedback-in #23(w330) -> ()
    n232 = feedback #24() -> (w331:bool)  [unwired: 1 in]
    n233 = feedback-in #24(w332) -> ()
    n234 = case shown="True" w331 {
      tunnel: w333 -> [_ w359]
      tunnel: w329 -> [_ w361]
      frame False {
      }
      frame True {
        w362 = 0 ("Timeout")
        n235 = Build Array (concatenate)(w359, w361) -> (w360:fxp<+/-,32,14>[])
        n236 = disable-structure shown="Default" {
          disable-tunnel: w359 -> [w364 _]
          frame condition #0 {
            n237 = Index Array(array=w364, index #1=2 ("index"), index #2=3 ("index")) -> (element #1=w369:fxp<+/-,32,14>, element #2=w368:fxp<+/-,32,14>)
            n238 = Build Array(w369, w368) -> (w365:fxp<+/-,32,14>[])
            n239 = xnode ("FIFO Method Node")("Element"=w365, "Timeout"=0) -> ()  [unwired: 1 in, 2 out]
          }
          frame condition #1 (active) {
            # "Quench OFF"
          }
        }
        n240 = xnode ("FIFO Method Node")("Element"=w360, "Timeout"=w362) -> ()  [unwired: 1 in, 2 out]
        n241 = xnode ("FIFO Method Node")("Element"=w359, "Timeout"=w362) -> ()  [unwired: 1 in, 2 out]
      }
    }
  }
  n242 = timed-loop {
    timing: w21 -> [_]
    timing-out: [_] -> w20
    stop <- _ stop-if-true
    n243 = xnode ("FIFO Method Node")("Timeout"=0) -> ("Element"=w375:u64, "Timed Out?"=w374:bool)  [unwired: 1 in, 1 out]
    n244 = feedback #25() -> (w373:u64)  [unwired: 1 in]
    n245 = feedback-in #25(w375) -> ()
    n246 = feedback #26() -> (w372:bool)  [unwired: 1 in]
    n247 = feedback-in #26(w374) -> ()
    n248 = call "HandleFIFOsetting.vi"("timed out"=w372, "Value"=w373) -> ()  [unwired: 10 in]
  }
  n249 = timed-loop {
    timing: w14 -> [_]
    timing-out: [_] -> w13
    stop <- _ stop-if-true
    n250 = xnode ("FIFO Method Node")("Timeout"=0) -> ("Element"=w382:u64, "Timed Out?"=w380:bool)  [unwired: 1 in, 1 out]
    n251 = feedback #27() -> (w381:u64)  [unwired: 1 in]
    n252 = feedback-in #27(w382) -> ()
    n253 = feedback #28() -> (w379:bool)  [unwired: 1 in]
    n254 = feedback-in #28(w380) -> ()
    n255 = call "HandleFeedForward.vi"("timed out"=w379, "Value"=w381) -> ()  [unwired: 10 in]
  }
  n256 = timed-loop {
    timing: w10 -> [_]
    timing-out: [_] -> w9
    stop <- _ stop-if-true
    n257 = Index Array(array="Simulated phase") -> (element=w386:fxp<+,64,64>)  [unwired: 1 in]
    n258 = call "SignalGenerator_x410.vi"("phase"=w386, "Reset"=FALSE) -> ("Cos"=w389:fxp<+/-,18,1>, "Sin"=w390:fxp<+/-,18,1>)  [unwired: 7 in, 1 out]
    n259 = local read "Mode"() -> (w388:T2)
    n260 = case shown="\"Simulated\"" w388 {
      tunnel: w390 -> [_ w394]
      tunnel: w389 -> [_ w393]
      frame "Real IO", Default {
      }
      frame "Simulated" {
        n261 = Bundle By Name(cluster=T7 {"I"=0.0, "Q"=0.0, "overflow"=FALSE} ("Element"), "I"=w394, "Q"=w393) -> (w392:T7)
        n262 = xnode ("FIFO Method Node")("Element"=w392, "Timeout"=0) -> ()  [unwired: 1 in, 2 out]
      }
    }
  }
  n263 = node-c288(w9) -> ()
  n264 = node-c288(w4) -> ()
  n265 = node-c288(w20) -> ()
  n266 = node-c288(w13) -> ()
  n267 = node-c288(w11) -> ()
  n268 = node-c288(w16) -> ()
  n269 = node-c288(w18) -> ()
